vi "RunOneTest.vi"(6 "ShowPanel? (f)":bool=TRUE, 7 ".tst file":path, 8 "Error Array In":errorcluster[](array[cluster]), 11 "TestTreeTags":string[](array[string])=["0_3_0_0_0_12_73_110_105_116_32_97_110_100_32_82_117_110_80_84_72_48_0_0_0_84_0_0_0_10_1_67_5_85_115_101_114_115_6_80_117_98_108_105_99_8_80_114_111_106_101_99_116_115_5_73_67_68_65_83_9_85_115_101_114_70_105_108_101_115_7_80_108_117_103_105_110_115_6_83_101_110_115_111_114_9_82_111_111_109_65_108_101_114_116_14_82_111_111_109_65_108_101_114_116_49_46_105_110_105_0_0_0_3_0_0_0_18_69_114_114_111_114_83_101_118_101_114_105_116_121_44_83_116_111_112_0_0_0_22_83_101_110_115_111_114_67_114_101_97_116_101_83_101_115_115_105_111_110_44_35_36_0_0_0_14_83_101_110_115_111_114_83_116_97_114_116_44_35_36", "0_3_0_0_0_12_73_110_105_116_32_97_110_100_32_82_117_110_80_84_72_48_0_0_0_98_0_0_0_10_1_67_5_85_115_101_114_115_6_80_117_98_108_105_99_8_80_114_111_106_101_99_116_115_5_73_67_68_65_83_9_85_115_101_114_70_105_108_101_115_7_80_108_117_103_105_110_115_6_83_101_110_115_111_114_28_83_105_101_109_101_110_115_32_68_105_103_105_116_97_108_32_69_110_101_114_103_121_32_77_101_116_101_114_9_83_68_69_77_48_46_105_110_105_0_0_0_3_0_0_0_18_69_114_114_111_114_83_101_118_101_114_105_116_121_44_83_116_111_112_0_0_0_22_83_101_110_115_111_114_67_114_101_97_116_101_83_101_115_115_105_111_110_44_35_36_0_0_0_14_83_101_110_115_111_114_83_116_97_114_116_44_35_36"]) -> (0 "ErrorArray Out":errorcluster[](array[cluster]), 1 "TDMS Log File":path)   [LabVIEW 2018]
uses:
  NistPluggableModules/TestClass/Test.lvclass
  NistPluggableModules/TestClass/Test.lvclass/Test.ctl
  NistPluggableModules/TestClass/Accessors/Read ModuleIDs.vi
  NistPluggableModules/TestClass/Accessors/Read ModuleList.vi
  <userlib>/_OpenG.lib/array/array.llb/Remove Duplicates from 1D Array (Path)__ogtk.vi
  <userlib>/NIST/NISTErrorLib/NISTErrorLib.lvlib
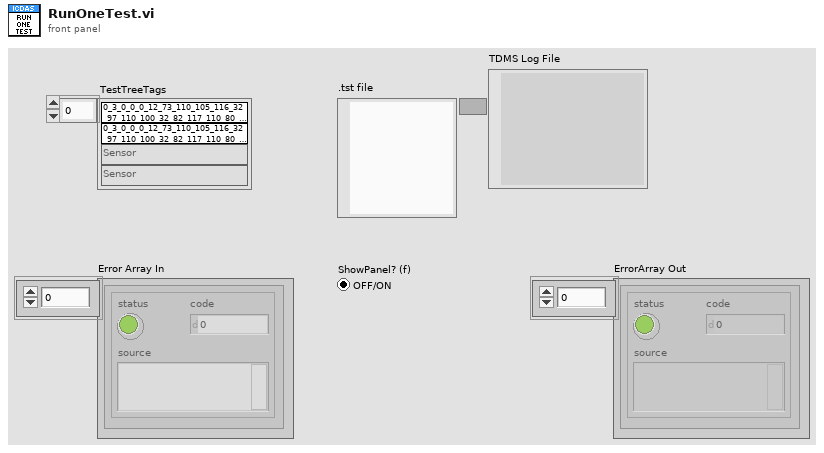
[diagram p1: front panel]
types:
  T1 = typedef "Plugin Tree Tag.ctl" = cluster{"ItemType":T2, "Name":string, "Path":path, "Script":string[]}
  T2 = typedef "Plugins Tree Item Type.ctl" = enum16{"Plugin", "Instrument", "INI File", "INI Script"}
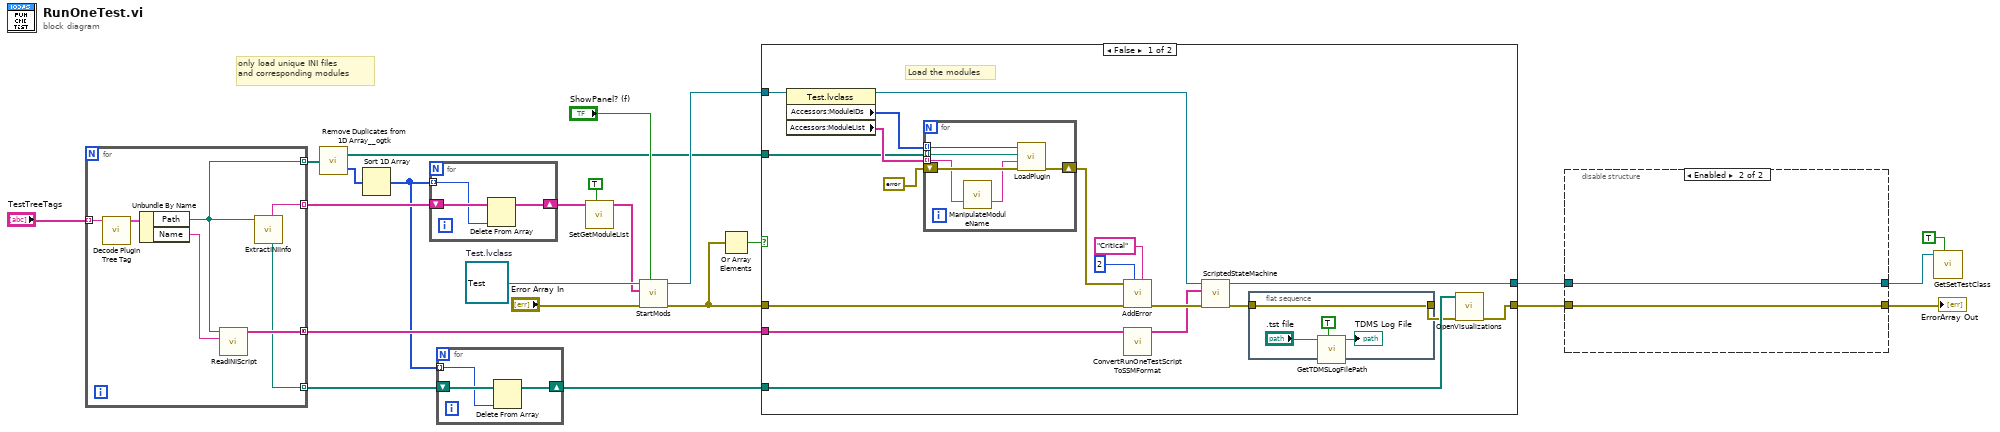
[diagram p0: block diagram]
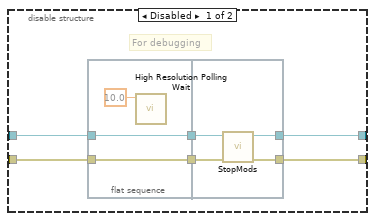
[diagram p3: hidden frame]
diagram:
  w23 = refnum<class "Test.lvclass"> refnum  # Test.lvclass
  # "only load unique INI files\nand corresponding modules"
  n1 = for {
    tunnel: "TestTreeTags" -> [w30] mode=indexing
    tunnel: [w27] -> w14 mode=indexing
    tunnel: [w28] -> w12 mode=indexing
    tunnel: [w26] -> w6 mode=concatenating
    tunnel: [w24] -> w3 mode=indexing
    n2 = call "Decode Plugin Tree Tag.vi"("Tag"=w30) -> ("Plugin Tree Tag"=w29:T1)  [unwired: 9 in, 1 out]
    n3 = Unbundle By Name(w29) -> ("Path"=w27:path, "Name"=w25:string)
    n4 = call "ReadINIScript.vi"("Script Name"=w25, "INI File Path"=w27) -> ("Script"=w26:string[])  [unwired: 6 in, 3 out]
    n5 = call "ExtractINIInfo.vi"("INI File Path"=w27) -> ("Visualization VI Path"=w24:path, "Module.INI File Name"=w28:string)  [unwired: 5 in, 4 out]
  }
  n6 = call-poly <userlib>:"Remove Duplicates from 1D Array__ogtk.vi"("Input Array"=w14) -> ("Output Array"=w13:path[], "indices of removed elements"=w15:i32[])
  n7 = Sort 1D Array(array=w15) -> (sorted array=w2:i32[])
  n8 = for {
    tunnel: w2 -> [w32] mode=indexing
    shift-right: [w31] -> w9
    shift-left: w12 -> [w33]
    n9 = Delete From Array(array=w33, index=w32) -> (array with subset deleted=w31:string[])  [unwired: 1 in, 1 out]
  }
  n10 = for {
    tunnel: w2 -> [w35] mode=indexing
    shift-right: [w34] -> w1
    shift-left: w3 -> [w36]
    n11 = Delete From Array(array=w36, index=w35) -> (array with subset deleted=w34:path[])  [unwired: 1 in, 1 out]
  }
  n12 = call "SetGetModuleList.vi"("Set? (F)"=TRUE, "ModuleList"=w9) -> ("ModuleList"=w8:string[])  [unwired: 9 in]
  n13 = call "StartMods.vi"("ShowPanel? (f)"="ShowPanel? (f)", "Error Array In"="Error Array In", "Module List"=w8, "Test.lvclass"=w23) -> ("Error Array Out"=w11:errorcluster[], "Test.lvclass"=w20:refnum<class "Test.lvclass">)  [unwired: 5 in, 1 out]
  n14 = Or Array Elements(Boolean array=w11) -> (logical OR=w21:bool)
  n15 = case shown="False" w21 {
    tunnel: w20 -> [w54 w66]
    tunnel: [w42 w66] -> w19
    tunnel: w13 -> [w51 _]
    tunnel: w11 -> [w39 w65]
    tunnel: [w41 w65] -> w10
    tunnel: w6 -> [w44 _]
    tunnel: w1 -> [w40 _]
    frame False {
      # "Load the modules"
      n16 = property class="Test.lvclass"(reference=w54) -> (reference out=w43:refnum<class "Test.lvclass">, "Accessors:ModuleIDs"=w53:i32[], "Accessors:ModuleList"=w52:string[])  [unwired: 1 in, 1 out]
      n17 = for {
        tunnel: w51 -> [w64] mode=indexing
        tunnel: w53 -> [w63] mode=indexing
        tunnel: w52 -> [w60] mode=indexing
        shift-right: [w62] -> w47
        shift-left: errorcluster {"status"=FALSE, "code"=0, "source"=""} ("error out") -> [w61]
        n18 = call "ManipulateModuleName.vi"("ModuleListSingleEntry"=w60) -> ("BeforeMatch:ModuleListSingleEntry"=w59:string)  [unwired: 9 in, 5 out]
        n19 = call "LoadPlugin.vi"("error in (no error)"=w61, "Module Name"=w59, "INI File Path"=w64, "Module ID"=w63) -> ("error out"=w62:errorcluster)  [unwired: 4 in, 3 out]
      }
      n20 = call <userlib>:"AddError.vi"("Severity"="Critical", "Priority"=u8 2, "ErrorArray In"=w39, "error in (no error)"=w47) -> ("ErrorArray Out"=w46:errorcluster[])  [unwired: 6 in, 1 out]
      n21 = call "ConvertRunOneTestScriptToSSMFormat.vi"("Script in"=w44) -> ("Script out"=w45:string[])  [unwired: 10 in]
      n22 = call "ScriptedStateMachine.vi"("ErrorArray"=w46, "script"=w45, "Test.lvclass"=w43) -> ("ErrorArray"=w38:errorcluster[], "Test.lvclass"=w42:refnum<class "Test.lvclass">)  [unwired: 6 in, 1 out]
      n23 = flat-sequence {
        tunnel: w38 -> [w56]
        tunnel: [w56] -> w37
        frame #0 {
          n24 = call "GetTDMSLogFilePath.vi"("Set? (F)"=TRUE, ".tst file"=".tst file") -> ("TDMS Log File Path"=→"TDMS Log File":path)  [unwired: 9 in]
        }
      }
      n25 = call "OpenVisualizations.vi"("ErrorArray in"=w37, "Visualization VI Paths"=w40) -> ("ErrorArray out"=w41:errorcluster[])  [unwired: 9 in]
    }
    frame True {
    }
  }
  n26 = disable-structure shown="Enabled" {
    disable-tunnel: w19 -> [w72 w81]
    disable-tunnel: w10 -> [w71 w80]
    disable-tunnel: [w70 w80] -> w17
    disable-tunnel: [w69 w81] -> w4
    frame Disabled {
      # "For debugging"
      n27 = flat-sequence {
        tunnel: w71 -> [w74]
        tunnel: w72 -> [w75]
        tunnel: [w75] -> w68
        tunnel: [w74] -> w67
        tunnel: [w77] -> w70
        tunnel: [w76] -> w69
        tunnel: w68 -> [w79]
        tunnel: w67 -> [w78]
        frame #0 {
          n28 = call <vilib>:"High Resolution Polling Wait.vi"("seconds to wait"=10.0) -> ()  [unwired: 10 in, 1 out]
        }
        frame #1 {
          n29 = call "StopMods.vi"("ErrorArray In"=w78, "Test.lvclass"=w79) -> ("ErrorArray Out"=w77:errorcluster[], "Test.lvclass"=w76:refnum<class "Test.lvclass">)  [unwired: 8 in]
        }
      }
    }
    frame Enabled {
    }
  }
  "ErrorArray Out" <- w17
  n30 = call "GetSetTestClass.vi"("Set"=TRUE, "Test.lvclass"=w4) -> ()  [unwired: 9 in, 1 out]
